vi "Headless Video Analyzer Get Timeout.vi"(1 "Status":T1) -> (0 "timeout":i32)   [LabVIEW 2018]
uses:
  Headless Video Analyzer Status STYP.ctl
  Classes/Video File/Video File.lvclass
  Classes/Video Frame/Video Frame.lvclass
  Classes/Message/Message.lvclass
  <vilib>/vision/Image Controls.llb/IMAQ Image.ctl
  Shared/Roughness Parameters STYP.ctl
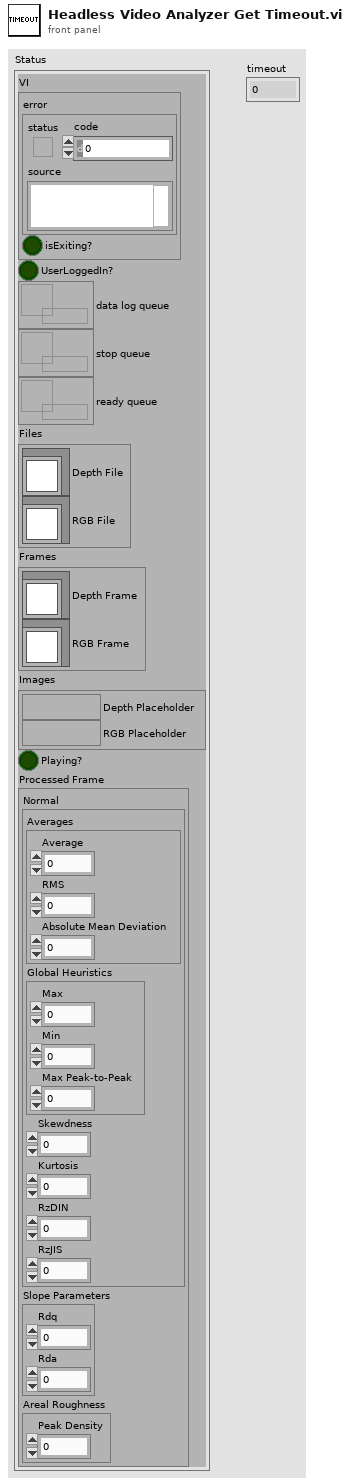
[diagram p1: front panel]
types:
  T1 = typedef "Headless Video Analyzer Status STYP.ctl" = cluster{"VI":cluster{"error":errorcluster, "isExiting?":bool}, "UserLoggedIn?":bool, "data log queue":refnum<queue>, "stop queue":refnum<queue>, "ready queue":refnum<queue>, "Files":cluster{"Depth File":refnum<class "Video File.lvclass">, "RGB File":refnum<class "Video File.lvclass">}, "Frames":cluster{"Depth Frame":refnum<class "Video Frame.lvclass">, "RGB Frame":refnum<class "Video Frame.lvclass">}, "Images":cluster{"Depth Placeholder":T2, "RGB Placeholder":T2}, "Playing?":bool, "Processed Frame":T3}
  T2 = typedef "IMAQ Image.ctl" = refnum<image>
  T3 = typedef "Roughness Parameters STYP.ctl" = cluster{"Normal":cluster{"Averages":cluster{"Average":dbl, "RMS":dbl, "Absolute Mean Deviation":dbl}, "Global Heuristics":cluster{"Max":dbl, "Min":dbl, "Max Peak-to-Peak":dbl}, "Skewdness":dbl, "Kurtosis":dbl, "RzDIN":dbl, "RzJIS":dbl}, "Slope Parameters":cluster{"Rdq":dbl, "Rda":dbl}, "Areal Roughness":cluster{"Peak Density":dbl}}
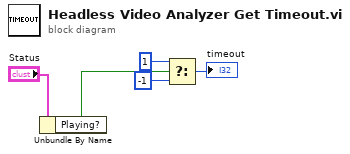
[diagram p0: block diagram]
diagram:
  n1 = Unbundle By Name("Status") -> ("Playing?"=w3:bool)
  n2 = Select(t=1, s=w3, f=-1) -> (s? t:f=→"timeout":i32)
